vi "Set Angle and Position.vi"(8 "error in (no error)":errorcluster, 9 "Angle":sgl(knob)=-0.03181185 scale=90.0..-90.0, 10 "Z":sgl=5.369775, 11 "XRay CArm in":refnum<class "XRay CArm.lvclass">=refnum) -> (0 "error out":errorcluster, 3 "XRay CArm out":refnum<class "XRay CArm.lvclass">)   [LabVIEW 2026, in "XRay CArm.lvclass"]
uses:
  XRay CArm.lvclass
  XRay CArm.lvclass/XRay CArm.ctl
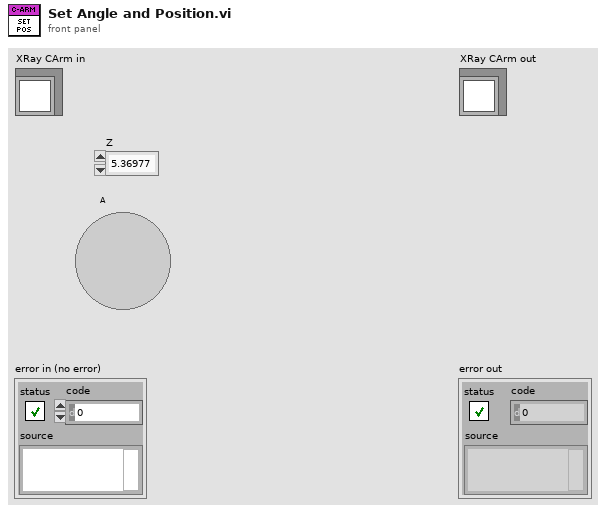
[diagram p1: front panel]
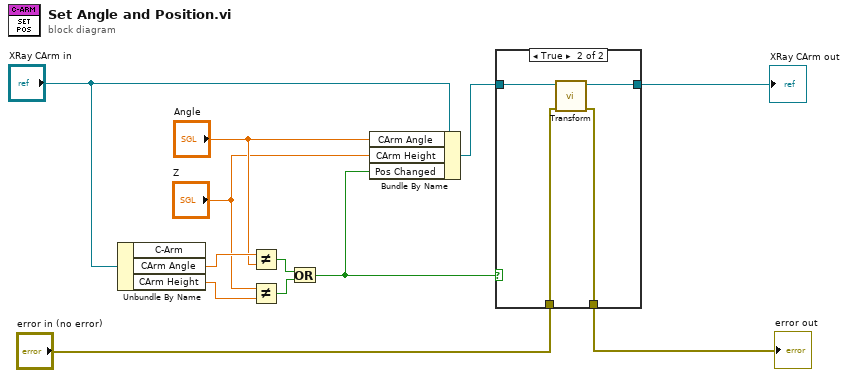
[diagram p0: block diagram]
diagram:
  n1 = Unbundle By Name("XRay CArm in") -> ("CArm Angle"=w12:sgl, "CArm Height"=w11:sgl)  [unwired: 1 out]
  n2 = Not Equal?(x=w12, y="Angle") -> (x != y?=w10:bool)
  n3 = Not Equal?(x="Z", y=w11) -> (x != y?=w9:bool)
  n4 = Or(x=w10, y=w9) -> (x .or. y?=w3:bool)
  n5 = Bundle By Name(cluster="XRay CArm in", "CArm Angle"="Angle", "CArm Height"="Z", "Pos Changed"=w3) -> (w5:refnum<class "XRay CArm.lvclass">)
  n6 = case shown="True" w3 {
    tunnel: w5 -> [w14 w18]
    tunnel: [w14 w17] -> w4
    tunnel: "error in (no error)" -> [w13 w16]
    tunnel: [w13 w15] -> w1
    frame False {
    }
    frame True {
      n7 = call-dynamic "Transform.vi"("error in (no error)"=w16, "XRay CArm in"=w18) -> ("error out"=w15:errorcluster, "XRay CArm out"=w17:refnum<class "XRay CArm.lvclass">)  [unwired: 8 in]
    }
  }
  "error out" <- w1
  "XRay CArm out" <- w4
